vi "Is DAA.vi"(8 "error in (no error)":errorcluster, 11 "Model in":refnum<class "Model.lvclass">) -> (0 "error out":errorcluster, 2 "IsDAA":bool, 3 "Model out":refnum<class "Model.lvclass">)   [LabVIEW 2016, in "Model.lvclass"]
uses:
  Model.lvclass
  Common_RT_FAILC/DataTypes/FATypes.ctl
  Model.lvclass/Model.ctl
  Common_RT_FAILC/RTFAILC.lvlib
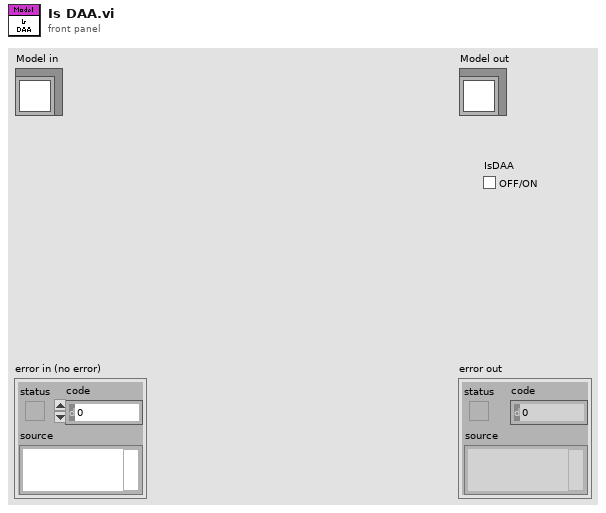
[diagram p1: front panel]
types:
  T1 = typedef "RTFAILC.lvlib/FATypes.ctl" = enum16{"SingleAxis", "LateralDualAxis", "CrossLateralDualAxis"}
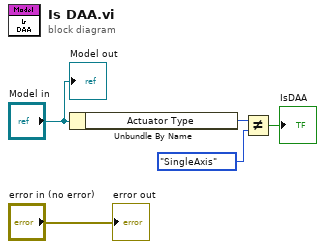
[diagram p0: block diagram]
diagram:
  n1 = Unbundle By Name("Model in") -> ("Actuator Type"=w5:T1)
  n2 = Not Equal?(x=w5, y=FATypes."SingleAxis") -> (x != y?=→"IsDAA":bool)
  "error out" <- "error in (no error)"
  "Model out" <- "Model in"
